vi "BalanceRudderSailSuggestion.vi"(6 "OLD Suggested Sail Setpoints":T1 {"MainSailSuggestion" min=0.0 max=1.0; "JibSailSuggestion" min=0.0 max=1.0}, 11 "ForceOnRudder":dbl) -> (3 "Suggested Sail Setpoints":T1 {"MainSailSuggestion" min=0.0 max=1.0; "JibSailSuggestion" min=0.0 max=1.0})   [LabVIEW 2013]
doc: "Takes in some measure of weather helm. This may be force on rudder, position of rudder (not straight when it should be straight), or even rate of turn when we should be going straight. The algorithm then decides how to adjust the sails to balance that weather helm.\n\nTHE SETTINGS COMING OUT OF THIS VI ARE RELATIVE. So if this VI outputs [-0.1, 0.1], it does not mean 'set the main to -0.1 and the jib to 0.1', it means 'adjust the main by 0.1 in and the jib by 0.1 out'.\n\nEric Schneider and Bonnie Ishiguro, Jan. 2014"
uses:
  Data/TypeDefs/Sail Set Suggestions.ctl
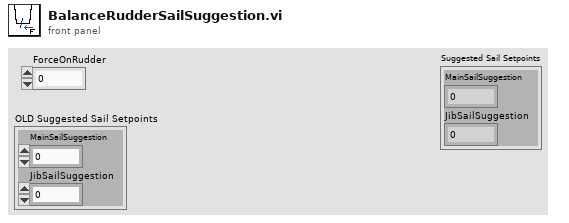
[diagram p1: front panel]
types:
  T1 = typedef "Sail Set Suggestions.ctl" = cluster{"MainSailSuggestion":dbl, "JibSailSuggestion":dbl}
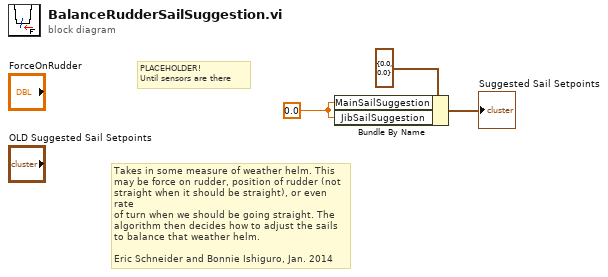
[diagram p0: block diagram]
diagram:
  w1 = 0.0 ("JibSailSuggestion")
  # "PLACEHOLDER!\nUntil sensors are there"
  # "Takes in some measure of weather helm. This\nmay be force on rudder, position of rudder (not\nstraight when it should be straight), or even rate\nof turn when we should be going straight. The\nalgorithm then decides how to adjust the sails\nto balance that weather helm.\n\nEric Schneider and Bonnie Ishiguro, Jan. 2014"
  n1 = Bundle By Name(cluster=T1 {"MainSailSuggestion"=0.0, "JibSailSuggestion"=0.0} ("output cluster"), "MainSailSuggestion"=w1, "JibSailSuggestion"=w1) -> (→"Suggested Sail Setpoints":T1)
